vi "pickKeeperTeam.vi"(8 "error in (no error)":errorcluster, 9 "RobotRef":refnum<class "Robot.lvclass">[](array[class]), 10 "number_of_robots":i32, 11 "Ally in":refnum<class "Ally.lvclass">) -> (0 "error out":errorcluster, 2 "RobotRef out":refnum<class "Robot.lvclass">[](array[class]), 3 "Ally out":refnum<class "Ally.lvclass">)   [LabVIEW 2018, in "Ally.lvclass"]
uses:
  Ally.lvclass
  C:/Users/nicolas.oliveira/roboime/SSL_AI/Team_class/Team.lvclass
  Robot_class/Robot.lvclass
  Team_class/Team.lvclass/Team.ctl
  Team_class/Write RobotRef.vi
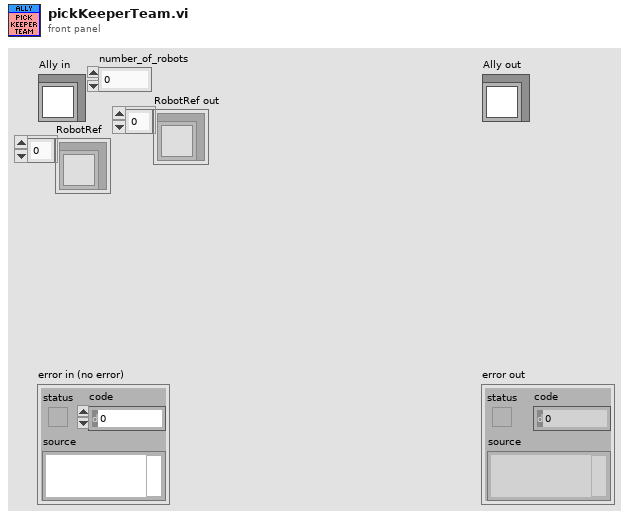
[diagram p1: front panel]
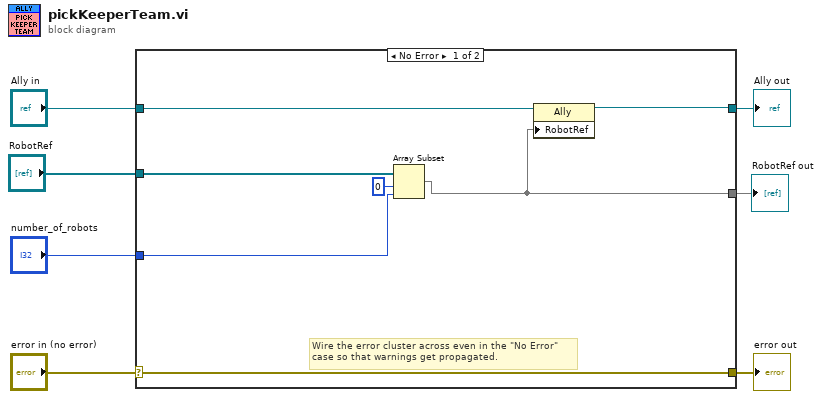
[diagram p0: block diagram]
diagram:
  n1 = case shown="No Error" "error in (no error)" {
    selector: "error in (no error)" -> [w14 w16]
    tunnel: [w14 w16] -> w6
    tunnel: [w10 w15] -> w4
    tunnel: "Ally in" -> [w11 w15]
    tunnel: "RobotRef" -> [w8 _]
    tunnel: "number_of_robots" -> [w12 _]
    tunnel: [w9 _] -> w1
    frame No Error {
      # "Wire the error cluster across even in the \"No Error\"\ncase so that warnings get propagated."
      n2 = Array Subset(array=w8, index=0, length=w12) -> (w9:refnum<class "Robot.lvclass">[])
      n3 = property class="Ally"(reference=w11, "RobotRef"=w9) -> (reference out=w10:refnum<class "Ally.lvclass">)  [unwired: 1 in, 1 out]
    }
    frame Error {
    }
  }
  "error out" <- w6
  "Ally out" <- w4
  "RobotRef out" <- w1
